vi "GrahamRobertsLab8.vi"() -> ()   [LabVIEW 2014]
panel:
  out "a\n b\nc":string[][](table)
  out "Table":string[][](table)
  out "Waveform Graph":dynamicdata(graph)
  out "Waveform Chart 2":dbl(graph)
  in  "stop":bool
  out "Waveform Chart":dynamicdata(graph)
  out "Numeric":dbl
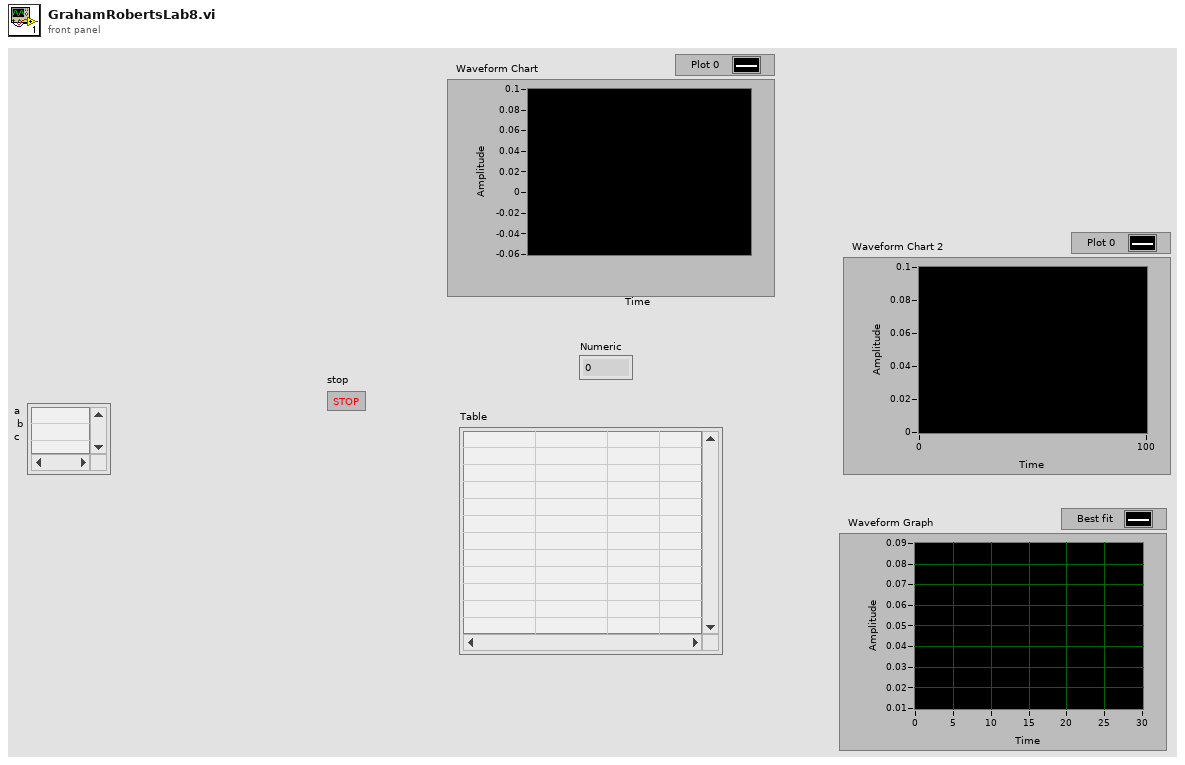
[diagram p1: front panel]
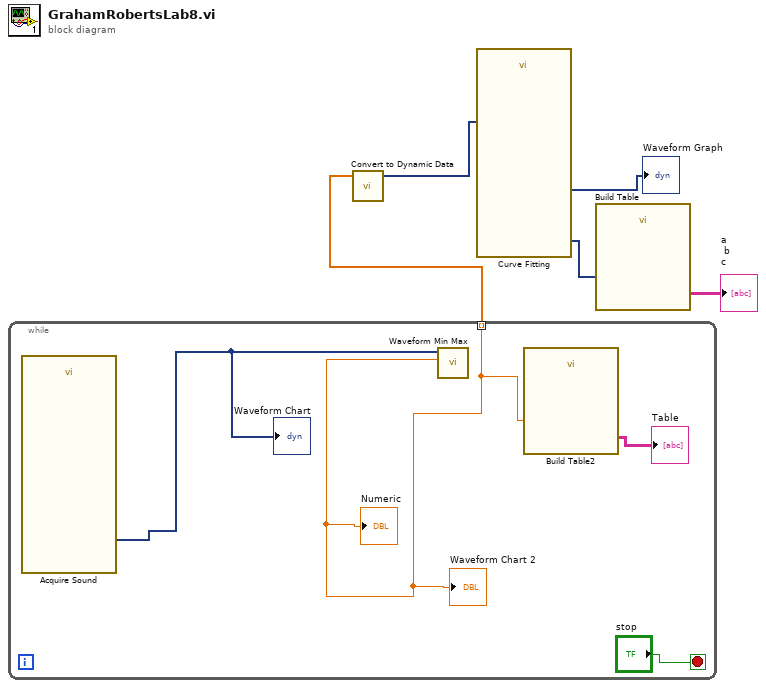
[diagram p0: block diagram]
diagram:
  n1 = while {
    tunnel: [w7] -> w5 mode=indexing
    stop <- "stop" stop-if-true
    n2 = call "Acquire Sound"() -> ("Data"=w9:dynamicdata)  [unwired: 18 in, 1 out]
    "Waveform Chart" <- w9
    n3 = call <vilib>:"Waveform Min Max.vi"("waveform in"=w9) -> ("Y max"=w7:dbl)  [unwired: 5 in, 5 out]
    "Numeric" <- w7
    "Waveform Chart 2" <- w7
    n4 = call "Build Table2"("Signals"=w7) -> ("Table"=→"Table":string[][])  [unwired: 4 in, 6 out]
  }
  n5 = call "Convert to Dynamic Data"("Array"=w5) -> ("Dynamic Data Type"=w4:dynamicdata)  [unwired: 3 in]
  n6 = call "Curve Fitting"("Signals"=w4) -> ("best fit"=→"Waveform Graph":dynamicdata, "non-linear coefficients"=w1:dynamicdata)  [unwired: 6 in, 3 out]
  n7 = call "Build Table"("Signals"=w1) -> ("Table"=→"a\n b\nc":string[][])  [unwired: 4 in, 6 out]
